vi "messageParser.vi"(9 "Completed Images In":u16[](array[numeric]), 10 "Input":string, 11 "Input Images":T1(array[cluster])) -> (1 "Completed Images Out":u16[](array[numeric]), 3 "OutputImages":T1(array[cluster]))   [LabVIEW 2014]
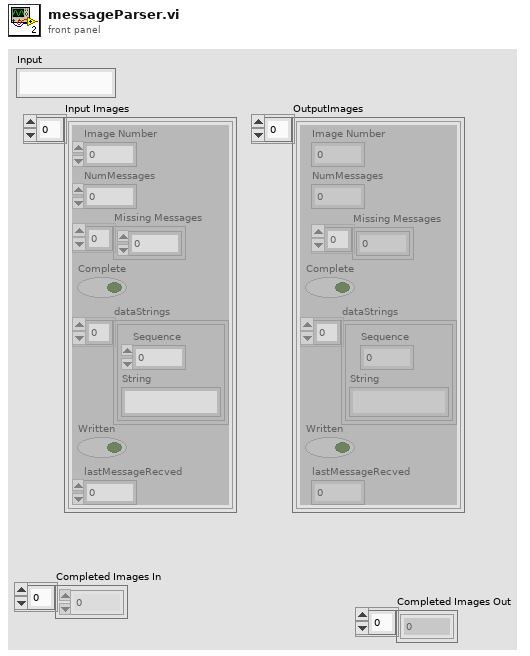
[diagram p1: front panel]
types:
  T1 = cluster{"Image Number":u16, "NumMessages":u16, "Missing Messages":u16[], "Complete":bool, "dataStrings":cluster{"Sequence":u16, "String":string}[], "Written":bool, "lastMessageRecved":u32}[]
  T2 = cluster{"Image Number":u16, "NumMessages":u16, "Missing Messages":u16[], "Complete":bool, "dataStrings":cluster{"Sequence":u16, "String":string}[], "Written":bool, "lastMessageRecved":u32}
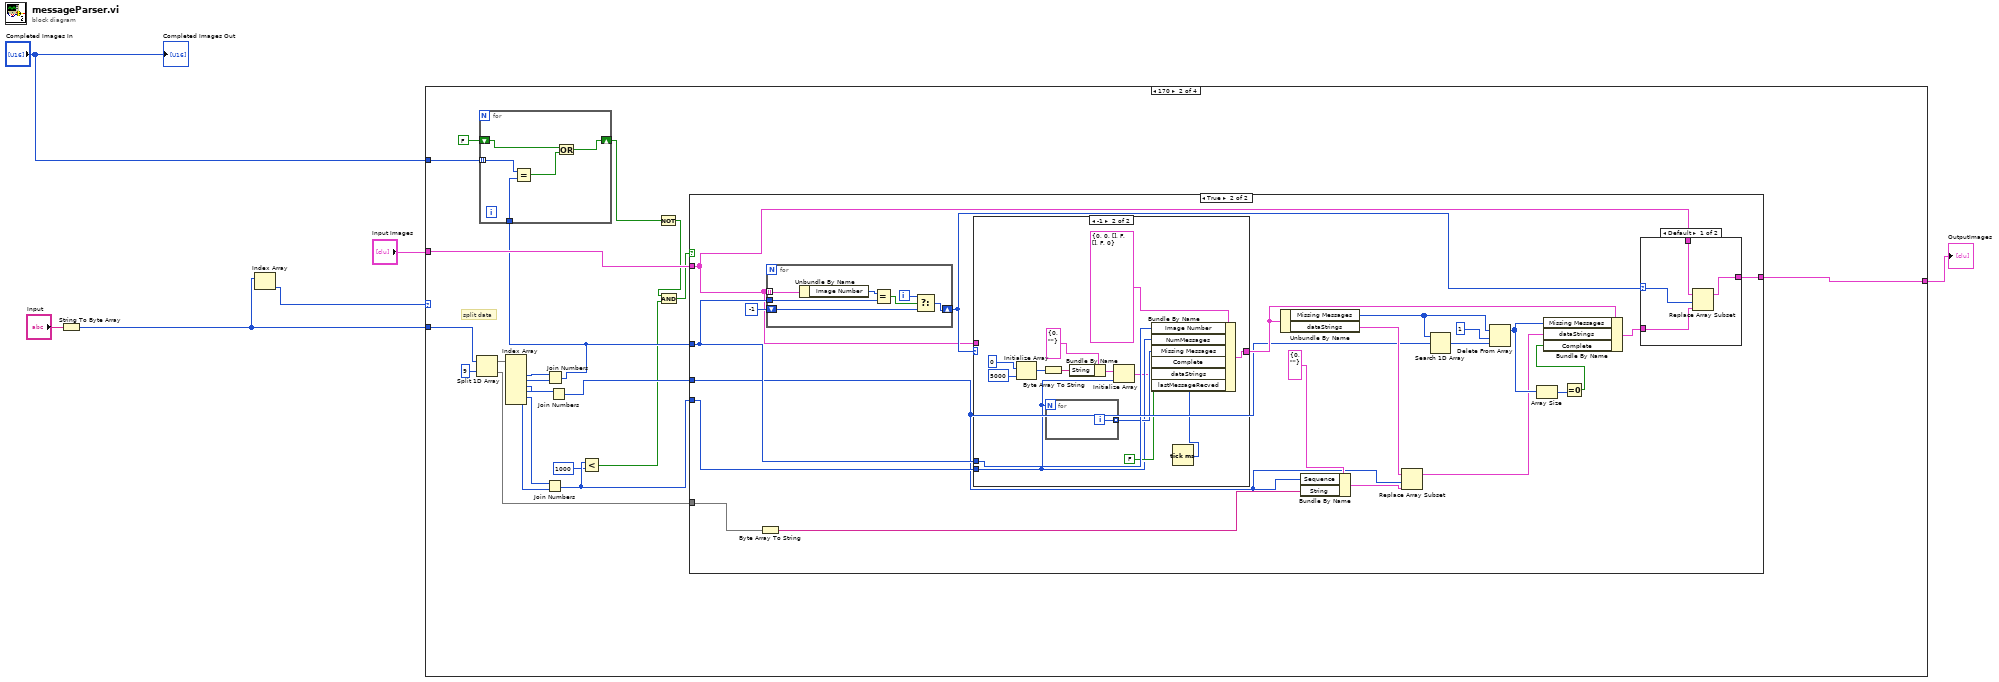
[diagram p0: block diagram]
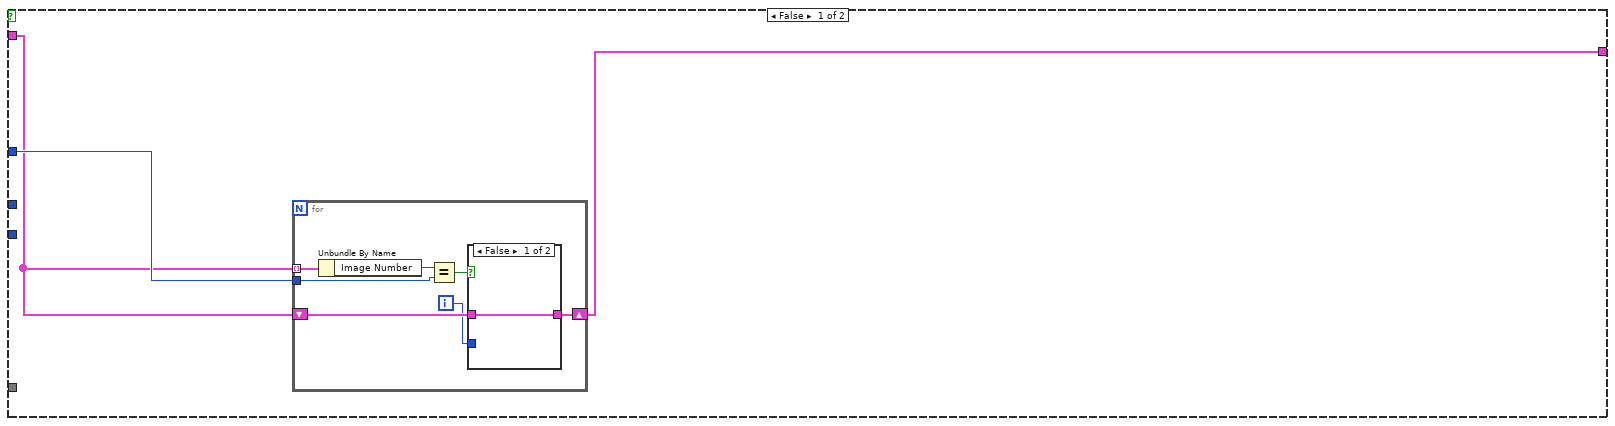
[diagram p3: hidden frame]
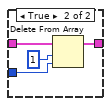
[diagram p4: hidden frame]
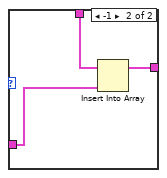
[diagram p5: hidden frame]
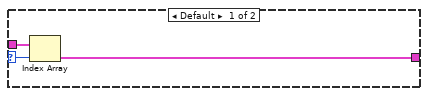
[diagram p6: hidden frame]
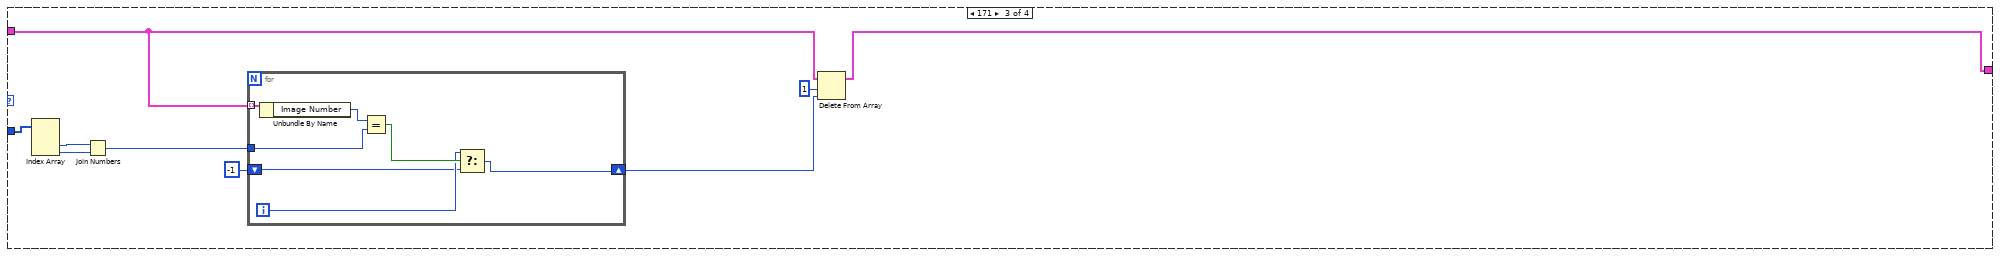
[diagram p7: hidden frame]
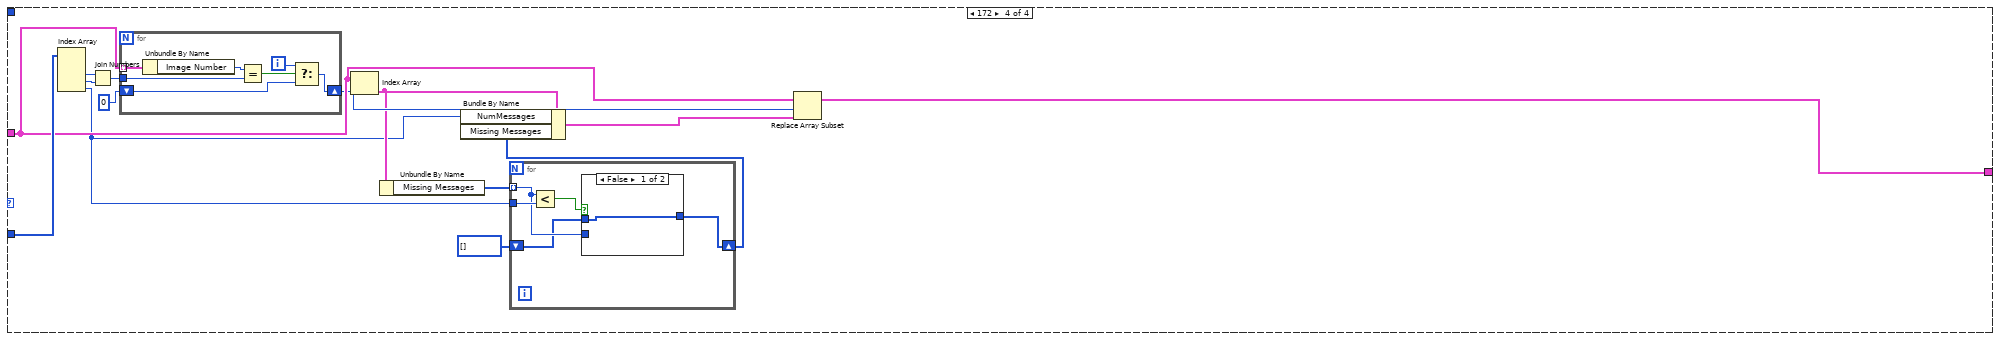
[diagram p8: hidden frame]
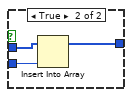
[diagram p9: hidden frame]
diagram:
  n1 = String To Byte Array(string="Input") -> (unsigned byte array=w2:u8[])
  n2 = Index Array(array=w2) -> (element=w1:u8)  [unwired: 1 in]
  n3 = case shown="170" w1 {
    tunnel: "Completed Images In" -> [_ w28 _ _]
    tunnel: [w7 w26 w109 w124] -> w4
    tunnel: "Input Images" -> [w7 w25 w110 w127]
    tunnel: w2 -> [_ w20 w105 w130]
    frame 0, Default {
    }
    frame 170 {
      # "split data"
      n4 = Split 1D Array(array=w20, index=9) -> (first subarray=w22:u8[], second subarray=w19:u8[])
      n5 = Index Array(array=w22) -> (element #2=w23:u8, element #3=w24:u8, element #4=w17:u8, element #5=w16:u8, element #6=w14:u8, element #7=w13:u8)  [unwired: 7 in, 1 out]
      n6 = Join Numbers(hi=w14, lo=w13) -> ((hi.lo)=w12:u16)
      n7 = Join Numbers(hi=w23, lo=w24) -> ((hi.lo)=w18:u16)
      n8 = for {
        tunnel: w28 -> [w34] mode=indexing
        tunnel: w18 -> [w33]
        shift-right: [w30] -> w27
        shift-left: FALSE -> [w31]
        n9 = Equal?(x=w34, y=w33) -> (x = y?=w32:bool)
        n10 = Or(x=w31, y=w32) -> (x .or. y?=w30:bool)
      }
      n11 = Join Numbers(hi=w17, lo=w16) -> ((hi.lo)=w15:u16)
      n12 = Less?(x=w12, y=u16 1000) -> (x < y?=w9:bool)
      n13 = Not(x=w27) -> (.not. x?=w10:bool)
      n14 = And(x=w10, y=w9) -> (x .and. y?=w8:bool)
      n15 = case shown="True" w8 {
        tunnel: w19 -> [_ w63]
        tunnel: w25 -> [w36 w59]
        tunnel: w18 -> [w37 w69]
        tunnel: w12 -> [_ w68]
        tunnel: w15 -> [_ w50]
        tunnel: [w35 w57] -> w26
        frame False {
          n16 = for {
            tunnel: w36 -> [w44] mode=indexing
            tunnel: w37 -> [w42]
            shift-right: [w39] -> w35
            shift-left: w36 -> [w40]
            i -> [w38]
            n17 = Unbundle By Name(w44) -> ("Image Number"=w43:u16)
            n18 = Equal?(x=w43, y=w42) -> (x = y?=w41:bool)
            n19 = case shown="False" w41 {
              tunnel: w40 -> [w45 w49]
              tunnel: [w45 w48] -> w39
              tunnel: w38 -> [_ w46]
              frame False {
              }
              frame True {
                n20 = Delete From Array(array=w49, length=1, index=w46) -> (array with subset deleted=w48:T1)  [unwired: 1 out]
              }
            }
          }
        }
        frame True {
          n21 = Byte Array To String(unsigned byte array=w63) -> (string=w61:string)
          n22 = for {
            tunnel: w59 -> [w102] mode=indexing
            tunnel: w69 -> [w100]
            shift-right: [w96] -> w60
            shift-left: -1 -> [w97]
            i -> [w98]
            n23 = Unbundle By Name(w102) -> ("Image Number"=w101:u16)
            n24 = Equal?(x=w101, y=w100) -> (x = y?=w99:bool)
            n25 = Select(t=w98, s=w99, f=w97) -> (s? t:f=w96:i32)
          }
          n26 = case shown="-1" w60 {
            selector: w60 -> [w80 _]
            tunnel: w59 -> [w79 _]
            tunnel: [w78 w91] -> w64
            tunnel: w69 -> [_ w94]
            tunnel: w68 -> [_ w89]
            frame Default {
              n27 = Index Array(array=w79, index=w80) -> (element=w78:T2)
            }
            frame -1 {
              n28 = Initialize Array(u8 0, 5000 ("dimension size")) -> (w85:u8[])
              n29 = Byte Array To String(unsigned byte array=w85) -> (string=w83:string)
              n30 = for {
                N: w89 -> [_]
                tunnel: [w95] -> w93 mode=indexing
                i -> [w95]
              }
              n31 = Bundle By Name(cluster=cluster{"Sequence":u16, "String":string} {"Sequence"=0, "String"=""} ("Cluster"), "String"=w83) -> (w82:cluster{"Sequence":u16, "String":string})
              n32 = Initialize Array(w82, w89) -> (w88:cluster{"Sequence":u16, "String":string}[])
              n33 = Tick Count (ms)() -> (millisecond timer value=w81:u32)
              n34 = Bundle By Name(cluster=T2 {"Image Number"=0, "NumMessages"=0, "Missing Messages"=[], "Complete"=FALSE, "dataStrings"=[], "Written"=FALSE, "lastMessageRecved"=0} ("Cluster"), "Image Number"=w94, "NumMessages"=w89, "Missing Messages"=w93, "Complete"=FALSE, "dataStrings"=w88, "lastMessageRecved"=w81) -> (w91:T2)
            }
          }
          n35 = Unbundle By Name(w64) -> ("Missing Messages"=w67:u16[], "dataStrings"=w53:cluster{"Sequence":u16, "String":string}[])
          n36 = Bundle By Name(cluster=cluster{"Sequence":u16, "String":string} {"Sequence"=0, "String"=""} ("new element/subarray"), "Sequence"=w50, "String"=w61) -> (w51:cluster{"Sequence":u16, "String":string})
          n37 = Replace Array Subset(array=w53, new element=w51, index=w50) -> (w52:cluster{"Sequence":u16, "String":string}[])
          n38 = Search 1D Array(1D array=w67, element=w50) -> (index of element=w66:i32)  [unwired: 1 in]
          n39 = Delete From Array(array=w67, length=1, index=w66) -> (array with subset deleted=w56:u16[])  [unwired: 1 out]
          n40 = Array Size(array=w56) -> (size(s)=w55:i32)
          n41 = Equal To 0?(x=w55) -> (x = 0?=w54:bool)
          n42 = Bundle By Name(cluster=w64, "Missing Messages"=w56, "dataStrings"=w52, "Complete"=w54) -> (w58:T2)
          n43 = case shown="Default" w60 {
            selector: w60 -> [w74 _]
            tunnel: w59 -> [w71 w75]
            tunnel: w58 -> [w73 w77]
            tunnel: [w72 w76] -> w57
            frame Default {
              n44 = Replace Array Subset(array=w71, new element=w73, index=w74) -> (w72:T1)
            }
            frame -1 {
              n45 = Insert Into Array(array=w75, new element=w77) -> (w76:T1)  [unwired: 1 in]
            }
          }
        }
      }
    }
    frame 171 {
      n46 = Index Array(array=w105) -> (element #2=w106:u8, element #3=w104:u8)  [unwired: 3 in, 1 out]
      n47 = Join Numbers(hi=w106, lo=w104) -> ((hi.lo)=w103:u16)
      n48 = for {
        tunnel: w110 -> [w118] mode=indexing
        shift-right: [w113] -> w107
        shift-left: -1 -> [w114]
        tunnel: w103 -> [w112]
        i -> [w115]
        n49 = Unbundle By Name(w118) -> ("Image Number"=w117:u16)
        n50 = Equal?(x=w117, y=w112) -> (x = y?=w116:bool)
        n51 = Select(t=w115, s=w116, f=w114) -> (s? t:f=w113:i32)
      }
      n52 = Delete From Array(array=w110, length=1, index=w107) -> (array with subset deleted=w109:T1)  [unwired: 1 out]
    }
    frame 172 {
      n53 = Index Array(array=w130) -> (element #2=w132:u8, element #3=w131:u8, element #4=w121:u8)  [unwired: 4 in, 1 out]
      n54 = Join Numbers(hi=w132, lo=w131) -> ((hi.lo)=w129:u16)
      n55 = for {
        tunnel: w127 -> [w148] mode=indexing
        tunnel: w129 -> [w146]
        shift-right: [w142] -> w126
        shift-left: 0 -> [w143]
        i -> [w144]
        n56 = Unbundle By Name(w148) -> ("Image Number"=w147:u16)
        n57 = Equal?(x=w147, y=w146) -> (x = y?=w145:bool)
        n58 = Select(t=w144, s=w145, f=w143) -> (s? t:f=w142:i32)
      }
      n59 = Index Array(array=w127, index=w126) -> (element=w123:T2)
      n60 = Unbundle By Name(w123) -> ("Missing Messages"=w122:u16[])
      n61 = for {
        tunnel: w122 -> [w135] mode=indexing
        tunnel: w121 -> [w137]
        shift-right: [w134] -> w119
        shift-left: u8[] [] -> [w133]
        n62 = Less?(x=w135, y=w137) -> (x < y?=w136:bool)
        n63 = case shown="False" w136 {
          tunnel: w135 -> [_ w141]
          tunnel: [w138 w140] -> w134
          tunnel: w133 -> [w138 w139]
          frame False {
          }
          frame True {
            n64 = Insert Into Array(array=w139, new element=w141) -> (w140:u8[])  [unwired: 1 in]
          }
        }
      }
      n65 = Bundle By Name(cluster=w123, "NumMessages"=w121, "Missing Messages"=w119) -> (w125:T2)
      n66 = Replace Array Subset(array=w127, new element=w125, index=w126) -> (w124:T1)
    }
  }
  "OutputImages" <- w4
  "Completed Images Out" <- "Completed Images In"
